vi "Init Hardware.vi"(8 "error in (no error)":errorcluster, 11 "CS580 Driver in":refnum<class "CS580 Driver.lvclass">) -> (0 "error out":errorcluster, 3 "CS580 Driver out":refnum<class "CS580 Driver.lvclass">)   [LabVIEW 2025, in "CS580 Driver.lvclass"]
uses:
  CS580 Driver.lvclass
  C:/GitHub/NHMFL_Core/Libraries/Instruments/VISA Instrument/VISA Instrument.lvclass
  C:/GitHub/NHMFL_Core/Libraries/Instruments/Instrument Driver/Instrument Driver.lvclass
  VISA Instrument/VISA Instrument.lvclass/VISA Instrument.ctl
  Instrument Driver/Instrument Driver.lvclass/Instrument Driver.ctl
  VISA Instrument/Read VISA resource.vi
  Instrument Driver/Read Recorder name.vi
  VISA Instrument/Write VISA resource.vi
  Instrument Driver/Write Channel names.vi
  Instrument Driver/Write Channel units.vi
  Simple VISA Reader/Simple VISA Reader Driver.lvclass
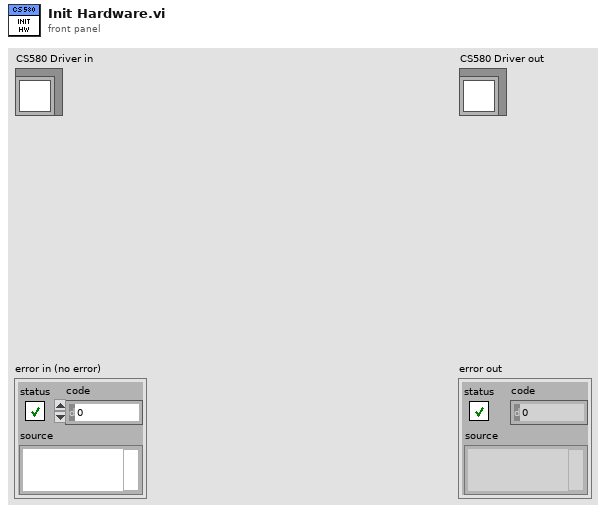
[diagram p1: front panel]
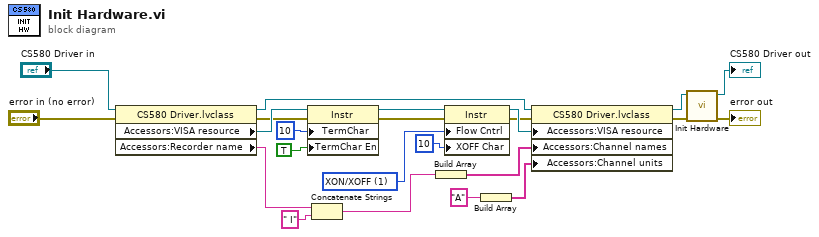
[diagram p0: block diagram]
diagram:
  w6 = u16 1 items=["None", "XON/XOFF", "RTS/CTS", "XON/XOFF & RTS/CTS", "DTR/DSR", "XON/XOFF & DTR/DSR"] ("Serial Settings:Flow Control")
  n1 = property class="CS580 Driver.lvclass"(reference="CS580 Driver in", error in="error in (no error)") -> (reference out=w21:refnum<class "CS580 Driver.lvclass">, error out=w7:errorcluster, "Accessors:VISA resource"=w10:refnum<visa-resource-name>, "Accessors:Recorder name"=w12:string)
  n2 = property class="Instr"(reference=w10, error in=w7, "TermChar"=u8 10 ("Message Based Settings:Termination Character"), "TermChar En"=TRUE ("Message Based Settings:Termination Character Enable")) -> (reference out=w4:refnum<visa-resource-name>, error out=w2:errorcluster)
  n3 = Concatenate Strings(w12, " I") -> (w18:string)
  n4 = Build Array(w18) -> (w11:string[])
  n5 = property class="Instr"(reference=w4, error in=w2, "Flow Cntrl"=w6, "XOFF Char"=u8 10 ("Serial Settings:Flow Control XOFF Character")) -> (reference out=w3:refnum<visa-resource-name>, error out=w1:errorcluster)
  n6 = Build Array("A") -> (w20:string[])
  n7 = property class="CS580 Driver.lvclass"(reference=w21, error in=w1, "Accessors:VISA resource"=w3, "Accessors:Channel names"=w11, "Accessors:Channel units"=w20) -> (reference out=w16:refnum<class "CS580 Driver.lvclass">, error out=w17:errorcluster)
  n8 = call-parent "Init Hardware.vi"("error in (no error)"=w17, "Instrument Driver in"=w16) -> ("error out"=→"error out":errorcluster, "Instrument Driver out"=→"CS580 Driver out":refnum<class "CS580 Driver.lvclass">)  [unwired: 8 in]
